vi "Get Message.vi"(8 "error in (no error)":errorcluster, 11 "Serial Communication in":refnum<class "Serial Communication.lvclass">) -> (0 "error out":errorcluster, 2 "Message":string, 3 "Serial Communication out":refnum<class "Serial Communication.lvclass">)   [LabVIEW 2018, in "Serial Communication.lvclass"]
uses:
  Serial Communication.lvclass
  Serial Communication.lvclass/Serial Communication.ctl
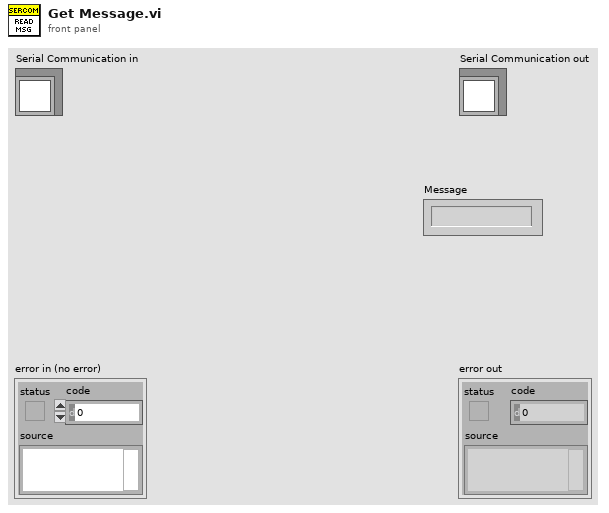
[diagram p1: front panel]
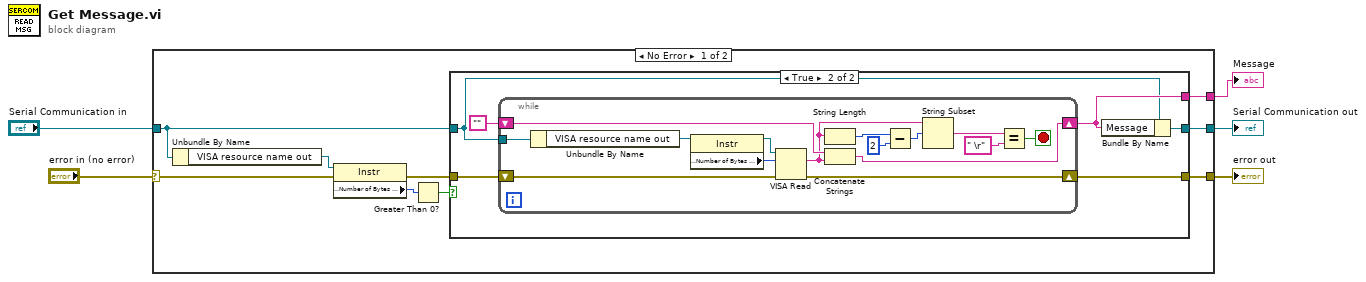
[diagram p0: block diagram]
diagram:
  n1 = case shown="No Error" "error in (no error)" {
    selector: "error in (no error)" -> [w14 w39]
    tunnel: [w12 w39] -> w4
    tunnel: [w9 w38] -> w2
    tunnel: "Serial Communication in" -> [w10 w38]
    tunnel: [w6 _] -> w1
    frame No Error {
      n2 = Unbundle By Name(w10) -> ("VISA resource name out"=w8:refnum<visa-resource-name>)
      n3 = property class="Instr"(reference=w8, error in=w14) -> (error out=w13:errorcluster, "Serial Settings:Number of Bytes at Serial Port"=w7:u32)  [unwired: 1 out]
      n4 = Greater Than 0?(x=w7) -> (x > 0?=w11:bool)
      n5 = case shown="True" w11 {
        tunnel: w13 -> [w16 w22]
        tunnel: [w16 w21] -> w12
        tunnel: w10 -> [w15 w19]
        tunnel: [w15 w18] -> w9
        tunnel: [_ w20] -> w6
        frame False {
        }
        frame True {
          n6 = while {
            tunnel: w19 -> [w35]
            shift-right: [w36] -> w21
            shift-left: w22 -> [w37]
            shift-right: [w31] -> w20
            shift-left: "" -> [w30]
            stop <- w23 stop-if-true
            n7 = Unbundle By Name(w35) -> ("VISA resource name out"=w34:refnum<visa-resource-name>)
            n8 = property class="Instr"(reference=w34) -> (reference out=w33:refnum<visa-resource-name>, "Serial Settings:Number of Bytes at Serial Port"=w32:u32)  [unwired: 1 in, 1 out]
            n9 = VISA Read(VISA resource name=w33, byte count=w32, error in (no error)=w37) -> (read buffer=w26:string, error out=w36:errorcluster)  [unwired: 2 out]
            n10 = String Length(string=w26) -> (length=w29:i32)
            n11 = Concatenate Strings(w30, w26) -> (w31:string)
            n12 = Subtract(x=w29, y=2) -> (x-y=w27:i32)
            n13 = String Subset(string=w26, offset (0)=w27) -> (substring=w25:string)  [unwired: 1 in]
            n14 = Equal?(x=w25, y=" \r") -> (x = y?=w23:bool)
          }
          n15 = Bundle By Name(cluster=w19, "Message"=w20) -> (w18:refnum<class "Serial Communication.lvclass">)
        }
      }
    }
    frame Error {
    }
  }
  "error out" <- w4
  "Serial Communication out" <- w2
  "Message" <- w1
